vi "Parse String.vi"(1 "String In":string) -> (0 "Array Out":string[](array[string]))   [LabVIEW 2013]
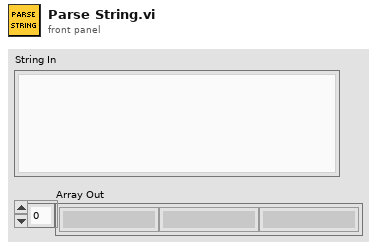
[diagram p1: front panel]
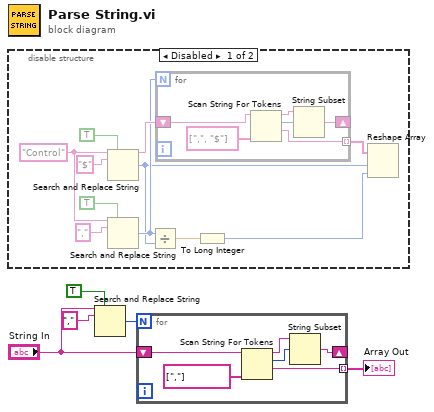
[diagram p0: block diagram]
diagram:
  n1 = disable-structure shown="Disabled" {
    frame Disabled {
      w6 = "Control" ("input string")
      n2 = Search and Replace String(replace all?=TRUE ("replace all? (F)"), input string=w6, search string="$") -> (result string=w12:string, number of replacements=w8:i32)  [unwired: 5 in, 2 out]
      n3 = Search and Replace String(replace all?=TRUE ("replace all? (F)"), input string=w6, search string=",") -> (number of replacements=w11:i32)  [unwired: 5 in, 3 out]
      n4 = Divide(x=w11, y=w8) -> (x/y=w10:dbl)
      n5 = for {
        N: w11 -> [_]
        shift-right: [w18] -> _
        shift-left: w12 -> [w19]
        tunnel: [w17] -> w7 mode=indexing
        n6 = Scan String For Tokens(6:string[] [",", "$"] ("delimiters (\\s,\\t,\\r,\\n)"), 9:w19) -> (1:w17:string, 2:w21:i32, 3:w20:string)  [unwired: 4 in, 1 out]
        n7 = String Subset(string=w20, offset (0)=w21) -> (substring=w18:string)  [unwired: 1 in]
      }
      n8 = To Long Integer(number=w10) -> (32bit integer=w9:i32)
      n9 = Reshape Array(w7, w8, w9) -> ()  [unwired: 1 out]
    }
    frame Enabled {
    }
  }
  n10 = Search and Replace String(replace all?=TRUE ("replace all? (F)"), input string="String In", search string=",") -> (number of replacements=w3:i32)  [unwired: 5 in, 3 out]
  n11 = for {
    N: w3 -> [_]
    tunnel: [w24] -> w1 mode=indexing
    shift-right: [w23] -> _
    shift-left: "String In" -> [w28]
    n12 = Scan String For Tokens(6:string[] [","] ("delimiters (\\s,\\t,\\r,\\n)"), 9:w28) -> (1:w24:string, 2:w25:i32, 3:w26:string)  [unwired: 4 in, 1 out]
    n13 = String Subset(string=w26, offset (0)=w25) -> (substring=w23:string)  [unwired: 1 in]
  }
  "Array Out" <- w1
